vi "Serial Communcation Devices GUID Lookup.vi"() -> ()   [LabVIEW 2017, in "Serial Communcation Devices Custom Device.lvlib"]
doc: "Use this Global VI to access the GUIDs assigned to the page resources of the Custom Device."
uses:
  Serial Communcation Devices Custom Device.lvlib
panel:
  in  "Channel Setting":string="43b76903-71cc-4e2b-b034-344d1b7f9646"
  in  "Custom Device":string="b73fe0e2-f08a-496c-bd7e-ac5d3d716b10"
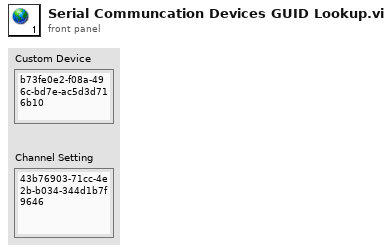
[diagram p1: front panel]
diagram:
